vi "test TCX read (installed 71).vi"() -> ()   [LabVIEW 2011] (continued)
ensions></Trackpoint><Trackpoint><Time>2008-03-03T23:23:27Z</Time><Position><LatitudeDegrees>35.882176</LatitudeDegrees><LongitudeDegrees>-78.947276</LongitudeDegrees></Position><AltitudeMeters>80.888</AltitudeMeters><DistanceMeters>20909.645</DistanceMeters><Cadence>83</Cadence><Extensions><TPX xmlns=\"http://www.garmin.com/xmlschemas/ActivityExtension/v2\"><Watts>156</Watts></TPX></Extensions></Trackpoint><Trackpoint><Time>2008-03-03T23:23:28Z</Time><Position><LatitudeDegrees>35.882253</LatitudeDegrees><LongitudeDegrees>-78.947252</LongitudeDegrees></Position><AltitudeMeters>80.888</AltitudeMeters><DistanceMeters>20918.570</DistanceMeters><Cadence>81</Cadence><Extensions><TPX xmlns=\"http://www.garmin.com/xmlschemas/ActivityExtension/v2\"><Watts>129</Watts></TPX></Extensions></Trackpoint><Trackpoint><Time>2008-03-03T23:23:29Z</Time><Position><LatitudeDegrees>35.882330</LatitudeDegrees><LongitudeDegrees>-78.947230</LongitudeDegrees></Position><AltitudeMeters>80.888</AltitudeMeters><DistanceMeters>20927.145</DistanceMeters><Cadence>80</Cadence><Extensions><TPX xmlns=\"http://www.garmin.com/xmlschemas/ActivityExtension/v2\"><Watts>133</Watts></TPX></Extensions></Trackpoint><Trackpoint><Time>2008-03-03T23:23:30Z</Time><Position><LatitudeDegrees>35.882405</LatitudeDegrees><LongitudeDegrees>-78.947209</LongitudeDegrees></Position><AltitudeMeters>81.369</AltitudeMeters><DistanceMeters>20935.766</DistanceMeters><Cadence>79</Cadence><Extensions><TPX xmlns=\"http://www.garmin.com/xmlschemas/ActivityExtension/v2\"><Watts>132</Watts></TPX></Extensions></Trackpoint><Trackpoint><Time>2008-03-03T23:23:31Z</Time><Position><LatitudeDegrees>35.882479</LatitudeDegrees><LongitudeDegrees>-78.947186</LongitudeDegrees></Position><AltitudeMeters>81.369</AltitudeMeters><DistanceMeters>20944.205</DistanceMeters><Cadence>78</Cadence><Extensions><TPX xmlns=\"http://www.garmin.com/xmlschemas/ActivityExtension/v2\"><Watts>147</Watts></TPX></Extensions></Trackpoint><Trackpoint><Time>2008-03-03T23:23:32Z</Time><Position><LatitudeDegrees>35.882553</LatitudeDegrees><LongitudeDegrees>-78.947165</LongitudeDegrees></Position><AltitudeMeters>81.369</AltitudeMeters><DistanceMeters>20952.598</DistanceMeters><Cadence>77</Cadence><Extensions><TPX xmlns=\"http://www.garmin.com/xmlschemas/ActivityExtension/v2\"><Watts>154</Watts></TPX></Extensions></Trackpoint><Trackpoint><Time>2008-03-03T23:23:33Z</Time><Position><LatitudeDegrees>35.882626</LatitudeDegrees><LongitudeDegrees>-78.947144</LongitudeDegrees></Position><AltitudeMeters>81.849</AltitudeMeters><DistanceMeters>20960.939</DistanceMeters><Cadence>77</Cadence><Extensions><TPX xmlns=\"http://www.garmin.com/xmlschemas/ActivityExtension/v2\"><Watts>162</Watts></TPX></Extensions></Trackpoint><Trackpoint><Time>2008-03-03T23:23:34Z</Time><Position><LatitudeDegrees>35.882699</LatitudeDegrees><LongitudeDegrees>-78.947123</LongitudeDegrees></Position><AltitudeMeters>81.849</AltitudeMeters><DistanceMeters>20969.234</DistanceMeters><Cadence>77</Cadence><Extensions><TPX xmlns=\"http://www.garmin.com/xmlschemas/ActivityExtension/v2\"><Watts>162</Watts></TPX></Extensions></Trackpoint><Trackpoint><Time>2008-03-03T23:23:35Z</Time><Position><LatitudeDegrees>35.882771</LatitudeDegrees><LongitudeDegrees>-78.947102</LongitudeDegrees></Position><AltitudeMeters>82.330</AltitudeMeters><DistanceMeters>20977.500</DistanceMeters><Cadence>77</Cadence><Extensions><TPX xmlns=\"http://www.garmin.com/xmlschemas/ActivityExtension/v2\"><Watts>163</Watts></TPX></Extensions></Trackpoint><Trackpoint><Time>2008-03-03T23:23:36Z</Time><Position><LatitudeDegrees>35.882844</LatitudeDegrees><LongitudeDegrees>-78.947082</LongitudeDegrees></Position><AltitudeMeters>82.330</AltitudeMeters><DistanceMeters>20985.758</DistanceMeters><Cadence>77</Cadence><Extensions><TPX xmlns=\"http://www.garmin.com/xmlschemas/ActivityExtension/v2\"><Watts>185</Watts></TPX></Extensions></Trackpoint><Trackpoint><Time>2008-03-03T23:23:37Z</Time><Position><LatitudeDegrees>35.882917</LatitudeDegrees><LongitudeDegrees>-78.947061</LongitudeDegrees></Position><AltitudeMeters>82.330</AltitudeMeters><DistanceMeters>20994.070</DistanceMeters><Cadence>77</Cadence><Extensions><TPX xmlns=\"http://www.garmin.com/xmlschemas/ActivityExtension/v2\"><Watts>195</Watts></TPX></Extensions></Trackpoint><Trackpoint><Time>2008-03-03T23:23:38Z</Time><Position><LatitudeDegrees>35.882990</LatitudeDegrees><LongitudeDegrees>-78.947042</LongitudeDegrees></Position><AltitudeMeters>82.330</AltitudeMeters><DistanceMeters>21002.367</DistanceMeters><Cadence>77</Cadence><Extensions><TPX xmlns=\"http://www.garmin.com/xmlschemas/ActivityExtension/v2\"><Watts>197</Watts></TPX></Extensions></Trackpoint><Trackpoint><Time>2008-03-03T23:23:39Z</Time><Position><LatitudeDegrees>35.883063</LatitudeDegrees><LongitudeDegrees>-78.947023</LongitudeDegrees></Position><AltitudeMeters>82.811</AltitudeMeters><DistanceMeters>21010.590</DistanceMeters><Cadence>77</Cadence><Extensions><TPX xmlns=\"http://www.garmin.com/xmlschemas/ActivityExtension/v2\"><Watts>196</Watts></TPX></Extensions></Trackpoint><Trackpoint><Time>2008-03-03T23:23:40Z</Time><Position><LatitudeDegrees>35.883135</LatitudeDegrees><LongitudeDegrees>-78.947001</LongitudeDegrees></Position><AltitudeMeters>82.811</AltitudeMeters><DistanceMeters>21018.857</DistanceMeters><Cadence>77</Cadence><Extensions><TPX xmlns=\"http://www.garmin.com/xmlschemas/ActivityExtension/v2\"><Watts>185</Watts></TPX></Extensions></Trackpoint><Trackpoint><Time>2008-03-03T23:23:41Z</Time><Position><LatitudeDegrees>35.883208</LatitudeDegrees><LongitudeDegrees>-78.946980</LongitudeDegrees></Position><AltitudeMeters>82.811</AltitudeMeters><DistanceMeters>21027.145</DistanceMeters><Cadence>76</Cadence><Extensions><TPX xmlns=\"http://www.garmin.com/xmlschemas/ActivityExtension/v2\"><Watts>181</Watts></TPX></Extensions></Trackpoint><Trackpoint><Time>2008-03-03T23:23:42Z</Time><Position><LatitudeDegrees>35.883280</LatitudeDegrees><LongitudeDegrees>-78.946958</LongitudeDegrees></Position><AltitudeMeters>82.811</AltitudeMeters><DistanceMeters>21035.389</DistanceMeters><Cadence>76</Cadence><Extensions><TPX xmlns=\"http://www.garmin.com/xmlschemas/ActivityExtension/v2\"><Watts>180</Watts></TPX></Extensions></Trackpoint><Trackpoint><Time>2008-03-03T23:23:43Z</Time><Position><LatitudeDegrees>35.883351</LatitudeDegrees><LongitudeDegrees>-78.946937</LongitudeDegrees></Position><AltitudeMeters>82.811</AltitudeMeters><DistanceMeters>21043.555</DistanceMeters><Cadence>76</Cadence><Extensions><TPX xmlns=\"http://www.garmin.com/xmlschemas/ActivityExtension/v2\"><Watts>159</Watts></TPX></Extensions></Trackpoint><Trackpoint><Time>2008-03-03T23:23:44Z</Time><Position><LatitudeDegrees>35.883423</LatitudeDegrees><LongitudeDegrees>-78.946915</LongitudeDegrees></Position><AltitudeMeters>83.291</AltitudeMeters><DistanceMeters>21051.729</DistanceMeters><Cadence>75</Cadence><Extensions><TPX xmlns=\"http://www.garmin.com/xmlschemas/ActivityExtension/v2\"><Watts>147</Watts></TPX></Extensions></Trackpoint><Trackpoint><Time>2008-03-03T23:23:45Z</Time><Position><LatitudeDegrees>35.883493</LatitudeDegrees><LongitudeDegrees>-78.946891</LongitudeDegrees></Position><AltitudeMeters>83.772</AltitudeMeters><DistanceMeters>21059.771</DistanceMeters><Cadence>74</Cadence><Extensions><TPX xmlns=\"http://www.garmin.com/xmlschemas/ActivityExtension/v2\"><Watts>148</Watts></TPX></Extensions></Trackpoint><Trackpoint><Time>2008-03-03T23:23:46Z</Time><Position><LatitudeDegrees>35.883561</LatitudeDegrees><LongitudeDegrees>-78.946866</LongitudeDegrees></Position><AltitudeMeters>83.291</AltitudeMeters><DistanceMeters>21067.736</DistanceMeters><Cadence>74</Cadence><Extensions><TPX xmlns=\"http://www.garmin.com/xmlschemas/ActivityExtension/v2\"><Watts>158</Watts></TPX></Extensions></Trackpoint><Trackpoint><Time>2008-03-03T23:23:47Z</Time><Position><LatitudeDegrees>35.883629</LatitudeDegrees><LongitudeDegrees>-78.946838</LongitudeDegrees></Position><AltitudeMeters>83.291</AltitudeMeters><DistanceMeters>21075.658</DistanceMeters><Cadence>74</Cadence><Extensions><TPX xmlns=\"http://www.garmin.com/xmlschemas/ActivityExtension/v2\"><Watts>159</Watts></TPX></Extensions></Trackpoint><Trackpoint><Time>2008-03-03T23:23:48Z</Time><Position><LatitudeDegrees>35.883696</LatitudeDegrees><LongitudeDegrees>-78.946808</LongitudeDegrees></Position><AltitudeMeters>83.772</AltitudeMeters><DistanceMeters>21083.572</DistanceMeters><Cadence>73</Cadence><Extensions><TPX xmlns=\"http://www.garmin.com/xmlschemas/ActivityExtension/v2\"><Watts>205</Watts></TPX></Extensions></Trackpoint><Trackpoint><Time>2008-03-03T23:23:49Z</Time><Position><LatitudeDegrees>35.883763</LatitudeDegrees><LongitudeDegrees>-78.946776</LongitudeDegrees></Position><AltitudeMeters>83.291</AltitudeMeters><DistanceMeters>21091.551</DistanceMeters><Cadence>74</Cadence><Extensions><TPX xmlns=\"http://www.garmin.com/xmlschemas/ActivityExtension/v2\"><Watts>230</Watts></TPX></Extensions></Trackpoint><Trackpoint><Time>2008-03-03T23:23:50Z</Time><Position><LatitudeDegrees>35.883829</LatitudeDegrees><LongitudeDegrees>-78.946741</LongitudeDegrees></Position><AltitudeMeters>83.291</AltitudeMeters><DistanceMeters>21099.539</DistanceMeters><Cadence>74</Cadence><Extensions><TPX xmlns=\"http://www.garmin.com/xmlschemas/ActivityExtension/v2\"><Watts>235</Watts></TPX></Extensions></Trackpoint><Trackpoint><Time>2008-03-03T23:23:51Z</Time><Position><LatitudeDegrees>35.883895</LatitudeDegrees><LongitudeDegrees>-78.946704</LongitudeDegrees></Position><AltitudeMeters>83.772</AltitudeMeters><DistanceMeters>21107.541</DistanceMeters><Cadence>74</Cadence><Extensions><TPX xmlns=\"http://www.garmin.com/xmlschemas/ActivityExtension/v2\"><Watts>234</Watts></TPX></Extensions></Trackpoint><Trackpoint><Time>2008-03-03T23:23:52Z</Time><Position><LatitudeDegrees>35.883959</LatitudeDegrees><LongitudeDegrees>-78.946664</LongitudeDegrees></Position><AltitudeMeters>84.253</AltitudeMeters><DistanceMeters>21115.559</DistanceMeters><Cadence>74</Cadence><Extensions><TPX xmlns=\"http://www.garmin.com/xmlschemas/ActivityExtension/v2\"><Watts>217</Watts></TPX></Extensions></Trackpoint><Trackpoint><Time>2008-03-03T23:23:53Z</Time><Position><LatitudeDegrees>35.884022</LatitudeDegrees><LongitudeDegrees>-78.946623</LongitudeDegrees></Position><AltitudeMeters>84.253</AltitudeMeters><DistanceMeters>21123.479</DistanceMeters><Cadence>74</Cadence><Extensions><TPX xmlns=\"http://www.garmin.com/xmlschemas/ActivityExtension/v2\"><Watts>205</Watts></TPX></Extensions></Trackpoint><Trackpoint><Time>2008-03-03T23:23:54Z</Time><Position><LatitudeDegrees>35.884085</LatitudeDegrees><LongitudeDegrees>-78.946579</LongitudeDegrees></Position><AltitudeMeters>84.733</AltitudeMeters><DistanceMeters>21131.467</DistanceMeters><Cadence>74</Cadence><Extensions><TPX xmlns=\"http://www.garmin.com/xmlschemas/ActivityExtension/v2\"><Watts>195</Watts></TPX></Extensions></Trackpoint><Trackpoint><Time>2008-03-03T23:23:55Z</Time><Position><LatitudeDegrees>35.884147</LatitudeDegrees><LongitudeDegrees>-78.946532</LongitudeDegrees></Position><AltitudeMeters>84.733</AltitudeMeters><DistanceMeters>21139.529</DistanceMeters><Cadence>74</Cadence><Extensions><TPX xmlns=\"http://www.garmin.com/xmlschemas/ActivityExtension/v2\"><Watts>184</Watts></TPX></Extensions></Trackpoint><Trackpoint><Time>2008-03-03T23:23:56Z</Time><Position><LatitudeDegrees>35.884208</LatitudeDegrees><LongitudeDegrees>-78.946484</LongitudeDegrees></Position><AltitudeMeters>85.214</AltitudeMeters><DistanceMeters>21147.596</DistanceMeters><Cadence>75</Cadence><Extensions><TPX xmlns=\"http://www.garmin.com/xmlschemas/ActivityExtension/v2\"><Watts>164</Watts></TPX></Extensions></Trackpoint><Trackpoint><Time>2008-03-03T23:23:57Z</Time><Position><LatitudeDegrees>35.884268</LatitudeDegrees><LongitudeDegrees>-78.946432</LongitudeDegrees></Position><AltitudeMeters>85.214</AltitudeMeters><DistanceMeters>21155.812</DistanceMeters><Cadence>76</Cadence><Extensions><TPX xmlns=\"http://www.garmin.com/xmlschemas/ActivityExtension/v2\"><Watts>145</Watts></TPX></Extensions></Trackpoint><Trackpoint><Time>2008-03-03T23:23:58Z</Time><Position><LatitudeDegrees>35.884328</LatitudeDegrees><LongitudeDegrees>-78.946376</LongitudeDegrees></Position><AltitudeMeters>85.214</AltitudeMeters><DistanceMeters>21164.123</DistanceMeters><Cadence>77</Cadence><Extensions><TPX xmlns=\"http://www.garmin.com/xmlschemas/ActivityExtension/v2\"><Watts>110</Watts></TPX></Extensions></Trackpoint><Trackpoint><Time>2008-03-03T23:23:59Z</Time><Position><LatitudeDegrees>35.884389</LatitudeDegrees><LongitudeDegrees>-78.946319</LongitudeDegrees></Position><AltitudeMeters>85.214</AltitudeMeters><DistanceMeters>21172.600</DistanceMeters><Cadence>77</Cadence><Extensions><TPX xmlns=\"http://www.garmin.com/xmlschemas/ActivityExtension/v2\"><Watts>111</Watts></TPX></Extensions></Trackpoint><Trackpoint><Time>2008-03-03T23:24:00Z</Time><Position><LatitudeDegrees>35.884449</LatitudeDegrees><LongitudeDegrees>-78.946261</LongitudeDegrees></Position><AltitudeMeters>85.214</AltitudeMeters><DistanceMeters>21181.143</DistanceMeters><Cadence>78</Cadence><Extensions><TPX xmlns=\"http://www.garmin.com/xmlschemas/ActivityExtension/v2\"><Watts>97</Watts></TPX></Extensions></Trackpoint><Trackpoint><Time>2008-03-03T23:24:01Z</Time><Position><LatitudeDegrees>35.884510</LatitudeDegrees><LongitudeDegrees>-78.946201</LongitudeDegrees></Position><AltitudeMeters>85.214</AltitudeMeters><DistanceMeters>21189.721</DistanceMeters><Cadence>80</Cadence><Extensions><TPX xmlns=\"http://www.garmin.com/xmlschemas/ActivityExtension/v2\"><Watts>98</Watts></TPX></Extensions></Trackpoint><Trackpoint><Time>2008-03-03T23:24:02Z</Time><Position><LatitudeDegrees>35.884571</LatitudeDegrees><LongitudeDegrees>-78.946138</LongitudeDegrees></Position><AltitudeMeters>84.733</AltitudeMeters><DistanceMeters>21198.600</DistanceMeters><Cadence>82</Cadence><Extensions><TPX xmlns=\"http://www.garmin.com/xmlschemas/ActivityExtension/v2\"><Watts>92</Watts></TPX></Extensions></Trackpoint><Trackpoint><Time>2008-03-03T23:24:03Z</Time><Position><LatitudeDegrees>35.884633</LatitudeDegrees><LongitudeDegrees>-78.946075</LongitudeDegrees></Position><AltitudeMeters>84.733</AltitudeMeters><DistanceMeters>21207.596</DistanceMeters><Cadence>85</Cadence><Extensions><TPX xmlns=\"http://www.garmin.com/xmlschemas/ActivityExtension/v2\"><Watts>83</Watts></TPX></Extensions></Trackpoint><Trackpoint><Time>2008-03-03T23:24:04Z</Time><Position><LatitudeDegrees>35.884699</LatitudeDegrees><LongitudeDegrees>-78.946010</LongitudeDegrees></Position><AltitudeMeters>84.253</AltitudeMeters><DistanceMeters>21216.910</DistanceMeters><Cadence>85</Cadence><Extensions><TPX xmlns=\"http://www.garmin.com/xmlschemas/ActivityExtension/v2\"><Watts>82</Watts></TPX></Extensions></Trackpoint><Trackpoint><Time>2008-03-03T23:24:05Z</Time><Position><LatitudeDegrees>35.884764</LatitudeDegrees><LongitudeDegrees>-78.945943</LongitudeDegrees></Position><AltitudeMeters>84.253</AltitudeMeters><DistanceMeters>21226.375</DistanceMeters><Cadence>87</Cadence><Extensions><TPX xmlns=\"http://www.garmin.com/xmlschemas/ActivityExtension/v2\"><Watts>76</Watts></TPX></Extensions></Trackpoint><Trackpoint><Time>2008-03-03T23:24:06Z</Time><Position><LatitudeDegrees>35.884828</LatitudeDegrees><LongitudeDegrees>-78.945874</LongitudeDegrees></Position><AltitudeMeters>84.253</AltitudeMeters><DistanceMeters>21235.848</DistanceMeters><Cadence>87</Cadence><Extensions><TPX xmlns=\"http://www.garmin.com/xmlschemas/ActivityExtension/v2\"><Watts>83</Watts></TPX></Extensions></Trackpoint><Trackpoint><Time>2008-03-03T23:24:07Z</Time><Position><LatitudeDegrees>35.884893</LatitudeDegrees><LongitudeDegrees>-78.945806</LongitudeDegrees></Position><AltitudeMeters>83.772</AltitudeMeters><DistanceMeters>21245.301</DistanceMeters><Cadence>87</Cadence><Extensions><TPX xmlns=\"http://www.garmin.com/xmlschemas/ActivityExtension/v2\"><Watts>95</Watts></TPX></Extensions></Trackpoint><Trackpoint><Time>2008-03-03T23:24:08Z</Time><Position><LatitudeDegrees>35.884958</LatitudeDegrees><LongitudeDegrees>-78.945738</LongitudeDegrees></Position><AltitudeMeters>83.291</AltitudeMeters><DistanceMeters>21254.760</DistanceMeters><Cadence>88</Cadence><Extensions><TPX xmlns=\"http://www.garmin.com/xmlschemas/ActivityExtension/v2\"><Watts>133</Watts></TPX></Extensions></Trackpoint><Trackpoint><Time>2008-03-03T23:24:09Z</Time><Position><LatitudeDegrees>35.885023</LatitudeDegrees><LongitudeDegrees>-78.945671</LongitudeDegrees></Position><AltitudeMeters>83.291</AltitudeMeters><DistanceMeters>21264.236</DistanceMeters><Cadence>88</Cadence><Extensions><TPX xmlns=\"http://www.garmin.com/xmlschemas/ActivityExtension/v2\"><Watts>134</Watts></TPX></Extensions></Trackpoint><Trackpoint><Time>2008-03-03T23:24:10Z</Time><Position><LatitudeDegrees>35.885089</LatitudeDegrees><LongitudeDegrees>-78.945603</LongitudeDegrees></Position><AltitudeMeters>83.772</AltitudeMeters><DistanceMeters>21273.727</DistanceMeters><Cadence>87</Cadence><Extensions><TPX xmlns=\"http://www.garmin.com/xmlschemas/ActivityExtension/v2\"><Watts>139</Watts></TPX></Extensions></Trackpoint><Trackpoint><Time>2008-03-03T23:24:11Z</Time><Position><LatitudeDegrees>35.885154</LatitudeDegrees><LongitudeDegrees>-78.945536</LongitudeDegrees></Position><AltitudeMeters>83.772</AltitudeMeters><DistanceMeters>21283.127</DistanceMeters><Cadence>86</Cadence><Extensions><TPX xmlns=\"http://www.garmin.com/xmlschemas/ActivityExtension/v2\"><Watts>133</Watts></TPX></Extensions></Trackpoint><Trackpoint><Time>2008-03-03T23:24:12Z</Time><Position><LatitudeDegrees>35.885218</LatitudeDegrees><LongitudeDegrees>-78.945470</LongitudeDegrees></Position><AltitudeMeters>83.772</AltitudeMeters><DistanceMeters>21292.441</DistanceMeters><Cadence>86</Cadence><Extensions><TPX xmlns=\"http://www.garmin.com/xmlschemas/ActivityExtension/v2\"><Watts>132</Watts></TPX></Extensions></Trackpoint><Trackpoint><Time>2008-03-03T23:24:13Z</Time><Position><LatitudeDegrees>35.885284</LatitudeDegrees><LongitudeDegrees>-78.945405</LongitudeDegrees></Position><AltitudeMeters>83.772</AltitudeMeters><DistanceMeters>21301.773</DistanceMeters><Cadence>87</Cadence><Extensions><TPX xmlns=\"http://www.garmin.com/xmlschemas/ActivityExtension/v2\"><Watts>184</Watts></TPX></Extensions></Trackpoint><Trackpoint><Time>2008-03-03T23:24:14Z</Time><Position><LatitudeDegrees>35.885350</LatitudeDegrees><LongitudeDegrees>-78.945340</LongitudeDegrees></Position><AltitudeMeters>83.772</AltitudeMeters><DistanceMeters>21311.172</DistanceMeters><Cadence>87</Cadence><Extensions><TPX xmlns=\"http://www.garmin.com/xmlschemas/ActivityExtension/v2\"><Watts>263</Watts></TPX></Extensions></Trackpoint><Trackpoint><Time>2008-03-03T23:24:15Z</Time><Position><LatitudeDegrees>35.885415</LatitudeDegrees><LongitudeDegrees>-78.945274</LongitudeDegrees></Position><AltitudeMeters>83.772</AltitudeMeters><DistanceMeters>21320.535</DistanceMeters><Cadence>86</Cadence><Extensions><TPX xmlns=\"http://www.garmin.com/xmlschemas/ActivityExtension/v2\"><Watts>270</Watts></TPX></Extensions></Trackpoint><Trackpoint><Time>2008-03-03T23:24:16Z</Time><Position><LatitudeDegrees>35.885479</LatitudeDegrees><LongitudeDegrees>-78.945208</LongitudeDegrees></Position><AltitudeMeters>84.253</AltitudeMeters><DistanceMeters>21329.799</DistanceMeters><Cadence>86</Cadence><Extensions><TPX xmlns=\"http://www.garmin.com/xmlschemas/ActivityExtension/v2\"><Watts>268</Watts></TPX></Extensions></Trackpoint><Trackpoint><Time>2008-03-03T23:24:17Z</Time><Position><LatitudeDegrees>35.885542</LatitudeDegrees><LongitudeDegrees>-78.945140</LongitudeDegrees></Position><AltitudeMeters>84.733</AltitudeMeters><DistanceMeters>21339.119</DistanceMeters><Cadence>86</Cadence><Extensions><TPX xmlns=\"http://www.garmin.com/xmlschemas/ActivityExtension/v2\"><Watts>258</Watts></TPX></Extensions></Trackpoint><Trackpoint><Time>2008-03-03T23:24:18Z</Time><Position><LatitudeDegrees>35.885605</LatitudeDegrees><LongitudeDegrees>-78.945072</LongitudeDegrees></Position><AltitudeMeters>84.733</AltitudeMeters><DistanceMeters>21348.438</DistanceMeters><Cadence>86</Cadence><Extensions><TPX xmlns=\"http://www.garmin.com/xmlschemas/ActivityExtension/v2\"><Watts>263</Watts></TPX></Extensions></Trackpoint><Trackpoint><Time>2008-03-03T23:24:19Z</Time><Position><LatitudeDegrees>35.885670</LatitudeDegrees><LongitudeDegrees>-78.945004</LongitudeDegrees></Position><AltitudeMeters>85.214</AltitudeMeters><DistanceMeters>21357.840</DistanceMeters><Cadence>86</Cadence><Extensions><TPX xmlns=\"http://www.garmin.com/xmlschemas/ActivityExtension/v2\"><Watts>263</Watts></TPX></Extensions></Trackpoint><Trackpoint><Time>2008-03-03T23:24:20Z</Time><Position><LatitudeDegrees>35.885735</LatitudeDegrees><LongitudeDegrees>-78.944938</LongitudeDegrees></Position><AltitudeMeters>85.695</AltitudeMeters><DistanceMeters>21367.240</DistanceMeters><Cadence>87</Cadence><Extensions><TPX xmlns=\"http://www.garmin.com/xmlschemas/ActivityExtension/v2\"><Watts>283</Watts></TPX></Extensions></Trackpoint><Trackpoint><Time>2008-03-03T23:24:21Z</Time><Position><LatitudeDegrees>35.885800</LatitudeDegrees><LongitudeDegrees>-78.944872</LongitudeDegrees></Position><AltitudeMeters>86.175</AltitudeMeters><DistanceMeters>21376.639</DistanceMeters><Cadence>86</Cadence><Extensions><TPX xmlns=\"http://www.garmin.com/xmlschemas/ActivityExtension/v2\"><Watts>281</Watts></TPX></Extensions></Trackpoint><Trackpoint><Time>2008-03-03T23:24:22Z</Time><Position><LatitudeDegrees>35.885866</LatitudeDegrees><LongitudeDegrees>-78.944809</LongitudeDegrees></Position><AltitudeMeters>86.175</AltitudeMeters><DistanceMeters>21385.852</DistanceMeters><Cadence>85</Cadence><Extensions><TPX xmlns=\"http://www.garmin.com/xmlschemas/ActivityExtension/v2\"><Watts>265</Watts></TPX></Extensions></Trackpoint><Trackpoint><Time>2008-03-03T23:24:23Z</Time><Position><LatitudeDegrees>35.885930</LatitudeDegrees><LongitudeDegrees>-78.944748</LongitudeDegrees></Position><AltitudeMeters>85.695</AltitudeMeters><DistanceMeters>21394.875</DistanceMeters><Cadence>83</Cadence><Extensions><TPX xmlns=\"http://www.garmin.com/xmlschemas/ActivityExtension/v2\"><Watts>180</Watts></TPX></Extensions></Trackpoint><Trackpoint><Time>2008-03-03T23:24:24Z</Time><Position><LatitudeDegrees>35.885996</LatitudeDegrees><LongitudeDegrees>-78.944689</LongitudeDegrees></Position><AltitudeMeters>85.695</AltitudeMeters><DistanceMeters>21403.871</DistanceMeters><Cadence>83</Cadence><Extensions><TPX xmlns=\"http://www.garmin.com/xmlschemas/ActivityExtension/v2\"><Watts>179</Watts></TPX></Extensions></Trackpoint><Trackpoint><Time>2008-03-03T23:24:25Z</Time><Position><LatitudeDegrees>35.886062</LatitudeDegrees><LongitudeDegrees>-78.944634</LongitudeDegrees></Position><AltitudeMeters>85.695</AltitudeMeters><DistanceMeters>21412.711</DistanceMeters><Cadence>81</Cadence><Extensions><TPX xmlns=\"http://www.garmin.com/xmlschemas/ActivityExtension/v2\"><Watts>164</Watts></TPX></Extensions></Trackpoint><Trackpoint><Time>2008-03-03T23:24:26Z</Time><Position><LatitudeDegrees>35.886128</LatitudeDegrees><LongitudeDegrees>-78.944583</LongitudeDegrees></Position><AltitudeMeters>85.695</AltitudeMeters><DistanceMeters>21421.385</DistanceMeters><Cadence>80</Cadence><Extensions><TPX xmlns=\"http://www.garmin.com/xmlschemas/ActivityExtension/v2\"><Watts>154</Watts></TPX></Extensions></Trackpoint><Trackpoint><Time>2008-03-03T23:24:27Z</Time><Position><LatitudeDegrees>35.886195</LatitudeDegrees><LongitudeDegrees>-78.944536</LongitudeDegrees></Position><AltitudeMeters>85.695</AltitudeMeters><DistanceMeters>21429.920</DistanceMeters><Cadence>78</Cadence><Extensions><TPX xmlns=\"http://www.garmin.com/xmlschemas/ActivityExtension/v2\"><Watts>153</Watts></TPX></Extensions></Trackpoint><Trackpoint><Time>2008-03-03T23:24:28Z</Time><Position><LatitudeDegrees>35.886263</LatitudeDegrees><LongitudeDegrees>-78.944493</LongitudeDegrees></Position><AltitudeMeters>85.695</AltitudeMeters><DistanceMeters>21438.398</DistanceMeters><Cadence>78</Cadence><Extensions><TPX xmlns=\"http://www.garmin.com/xmlschemas/ActivityExtension/v2\"><Watts>150</Watts></TPX></Extensions></Trackpoint><Trackpoint><Time>2008-03-03T23:24:29Z</Time><Position><LatitudeDegrees>35.886333</LatitudeDegrees><LongitudeDegrees>-78.944455</LongitudeDegrees></Position><AltitudeMeters>85.695</AltitudeMeters><DistanceMeters>21446.896</DistanceMeters><Cadence>79</Cadence><Extensions><TPX xmlns=\"http://www.garmin.com/xmlschemas/ActivityExtension/v2\"><Watts>130</Watts></TPX></Extensions></Trackpoint><Trackpoint><Time>2008-03-03T23:24:30Z</Time><Position><LatitudeDegrees>35.886404</LatitudeDegrees><LongitudeDegrees>-78.944421</LongitudeDegrees></Position><AltitudeMeters>86.175</AltitudeMeters><DistanceMeters>21455.379</DistanceMeters><Cadence>78</Cadence><Extensions><TPX xmlns=\"http://www.garmin.com/xmlschemas/ActivityExtension/v2\"><Watts>114</Watts></TPX></Extensions></Trackpoint><Trackpoint><Time>2008-03-03T23:24:31Z</Time><Position><LatitudeDegrees>35.886477</LatitudeDegrees><LongitudeDegrees>-78.944391</LongitudeDegrees></Position><AltitudeMeters>85.695</AltitudeMeters><DistanceMeters>21463.840</DistanceMeters><Cadence>78</Cadence><Extensions><TPX xmlns=\"http://www.garmin.com/xmlschemas/ActivityExtension/v2\"><Watts>103</Watts></TPX></Extensions></Trackpoint><Trackpoint><Time>2008-03-03T23:24:32Z</Time><Position><LatitudeDegrees>35.886551</LatitudeDegrees><LongitudeDegrees>-78.944364</LongitudeDegrees></Position><AltitudeMeters>85.695</AltitudeMeters><DistanceMeters>21472.439</DistanceMeters><Cadence>79</Cadence><Extensions><TPX xmlns=\"http://www.garmin.com/xmlschemas/ActivityExtension/v2\"><Watts>103</Watts></TPX></Extensions></Trackpoint><Trackpoint><Time>2008-03-03T23:24:33Z</Time><Position><LatitudeDegrees>35.886626</LatitudeDegrees><LongitudeDegrees>-78.944337</LongitudeDegrees></Position><AltitudeMeters>85.214</AltitudeMeters><DistanceMeters>21481.201</DistanceMeters><Cadence>72</Cadence><Extensions><TPX xmlns=\"http://www.garmin.com/xmlschemas/ActivityExtension/v2\"><Watts>97</Watts></TPX></Extensions></Trackpoint><Trackpoint><Time>2008-03-03T23:24:34Z</Time><Position><LatitudeDegrees>35.886704</LatitudeDegrees><LongitudeDegrees>-78.944310</LongitudeDegrees></Position><AltitudeMeters>85.214</AltitudeMeters><DistanceMeters>21490.156</DistanceMeters><Cadence>74</Cadence><Extensions><TPX xmlns=\"http://www.garmin.com/xmlschemas/ActivityExtension/v2\"><Watts>113</Watts></TPX></Extensions></Trackpoint><Trackpoint><Time>2008-03-03T23:24:35Z</Time><Position><LatitudeDegrees>35.886784</LatitudeDegrees><LongitudeDegrees>-78.944284</LongitudeDegrees></Position><AltitudeMeters>85.214</AltitudeMeters><DistanceMeters>21499.391</DistanceMeters><Cadence>76</Cadence><Extensions><TPX xmlns=\"http://www.garmin.com/xmlschemas/ActivityExtension/v2\"><Watts>114</Watts></TPX></Extensions></Trackpoint><Trackpoint><Time>2008-03-03T23:24:36Z</Time><Position><LatitudeDegrees>35.886867</LatitudeDegrees><LongitudeDegrees>-78.944256</LongitudeDegrees></Position><AltitudeMeters>84.733</AltitudeMeters><DistanceMeters>21508.889</DistanceMeters><Cadence>78</Cadence><Extensions><TPX xmlns=\"http://www.garmin.com/xmlschemas/ActivityExtension/v2\"><Watts>115</Watts></TPX></Extensions></Trackpoint><Trackpoint><Time>2008-03-03T23:24:37Z</Time><Position><LatitudeDegrees>35.886951</LatitudeDegrees><LongitudeDegrees>-78.944226</LongitudeDegrees></Position><AltitudeMeters>84.733</AltitudeMeters><DistanceMeters>21518.637</DistanceMeters><Cadence>67</Cadence><Extensions><TPX xmlns=\"http://www.garmin.com/xmlschemas/ActivityExtension/v2\"><Watts>77</Watts></TPX></Extensions></Trackpoint><Trackpoint><Time>2008-03-03T23:24:38Z</Time><Position><LatitudeDegrees>35.887037</LatitudeDegrees><LongitudeDegrees>-78.944197</LongitudeDegrees></Position><AltitudeMeters>84.733</AltitudeMeters><DistanceMeters>21528.494</DistanceMeters><Cadence>67</Cadence><Extensions><TPX xmlns=\"http://www.garmin.com/xmlschemas/ActivityExtension/v2\"><Watts>78</Watts></TPX></Extensions></Trackpoint><Trackpoint><Time>2008-03-03T23:24:39Z</Time><Position><LatitudeDegrees>35.887126</LatitudeDegrees><LongitudeDegrees>-78.944186</LongitudeDegrees></Position><AltitudeMeters>84.733</AltitudeMeters><DistanceMeters>21538.449</DistanceMeters><Cadence>61</Cadence><Extensions><TPX xmlns=\"http://www.garmin.com/xmlschemas/ActivityExtension/v2\"><Watts>69</Watts></TPX></Extensions></Trackpoint><Trackpoint><Time>2008-03-03T23:24:40Z</Time><Position><LatitudeDegrees>35.887223</LatitudeDegrees><LongitudeDegrees>-78.944237</LongitudeDegrees></Position><AltitudeMeters>84.733</AltitudeMeters><DistanceMeters>21550.215</DistanceMeters><Cadence>61</Cadence><Extensions><TPX xmlns=\"http://www.garmin.com/xmlschemas/ActivityExtension/v2\"><Watts>69</Watts></TPX></Extensions></Trackpoint><Trackpoint><Time>2008-03-03T23:24:41Z</Time><Position><LatitudeDegrees>35.887305</LatitudeDegrees><LongitudeDegrees>-78.944319</LongitudeDegrees></Position><AltitudeMeters>84.253</AltitudeMeters><DistanceMeters>21561.879</DistanceMeters><Cadence>65</Cadence><Extensions><TPX xmlns=\"http://www.garmin.com/xmlschemas/ActivityExtension/v2\"><Watts>92</Watts></TPX></Extensions></Trackpoint><Trackpoint><Time>2008-03-03T23:24:42Z</Time><Position><LatitudeDegrees>35.887353</LatitudeDegrees><LongitudeDegrees>-78.944435</LongitudeDegrees></Position><AltitudeMeters>84.253</AltitudeMeters><DistanceMeters>21573.764</DistanceMeters><Cadence>66</Cadence><Extensions><TPX xmlns=\"http://www.garmin.com/xmlschemas/ActivityExtension/v2\"><Watts>111</Watts></TPX></Extensions></Trackpoint><Trackpoint><Time>2008-03-03T23:24:43Z</Time><Position><LatitudeDegrees>35.887385</LatitudeDegrees><LongitudeDegrees>-78.944552</LongitudeDegrees></Position><AltitudeMeters>82.811</AltitudeMeters><DistanceMeters>21584.902</DistanceMeters><Cadence>66</Cadence><Extensions><TPX xmlns=\"http://www.garmin.com/xmlschemas/ActivityExtension/v2\"><Watts>154</Watts></TPX></Extensions></Trackpoint><Trackpoint><Time>2008-03-03T23:24:44Z</Time><Position><LatitudeDegrees>35.887402</LatitudeDegrees><LongitudeDegrees>-78.944677</LongitudeDegrees></Position><AltitudeMeters>82.811</AltitudeMeters><DistanceMeters>21596.406</DistanceMeters><Cadence>69</Cadence><Extensions><TPX xmlns=\"http://www.garmin.com/xmlschemas/ActivityExtension/v2\"><Watts>230</Watts></TPX></Extensions></Trackpoint><Trackpoint><Time>2008-03-03T23:24:45Z</Time><Position><LatitudeDegrees>35.887414</LatitudeDegrees><LongitudeDegrees>-78.944808</LongitudeDegrees></Position><AltitudeMeters>83.291</AltitudeMeters><DistanceMeters>21608.266</DistanceMeters><Cadence>71</Cadence><Extensions><TPX xmlns=\"http://www.garmin.com/xmlschemas/ActivityExtension/v2\"><Watts>300</Watts></TPX></Extensions></Trackpoint><Trackpoint><Time>2008-03-03T23:24:46Z</Time><Position><LatitudeDegrees>35.887423</LatitudeDegrees><LongitudeDegrees>-78.944941</LongitudeDegrees></Position><AltitudeMeters>82.330</AltitudeMeters><DistanceMeters>21620.381</DistanceMeters><Cadence>72</Cadence><Extensions><TPX xmlns=\"http://www.garmin.com/xmlschemas/ActivityExtension/v2\"><Watts>336</Watts></TPX></Extensions></Trackpoint><Trackpoint><Time>2008-03-03T23:24:47Z</Time><Position><LatitudeDegrees>35.887426</LatitudeDegrees><LongitudeDegrees>-78.945076</LongitudeDegrees></Position><AltitudeMeters>81.849</AltitudeMeters><DistanceMeters>21632.525</DistanceMeters><Cadence>72</Cadence><Extensions><TPX xmlns=\"http://www.garmin.com/xmlschemas/ActivityExtension/v2\"><Watts>423</Watts></TPX></Extensions></Trackpoint><Trackpoint><Time>2008-03-03T23:24:48Z</Time><Position><LatitudeDegrees>35.887433</LatitudeDegrees><LongitudeDegrees>-78.945212</LongitudeDegrees></Position><AltitudeMeters>82.330</AltitudeMeters><DistanceMeters>21644.840</DistanceMeters><Cadence>72</Cadence><Extensions><TPX xmlns=\"http://www.garmin.com/xmlschemas/ActivityExtension/v2\"><Watts>418</Watts></TPX></Extensions></Trackpoint><Trackpoint><Time>2008-03-03T23:24:49Z</Time><Position><LatitudeDegrees>35.887438</LatitudeDegrees><LongitudeDegrees>-78.945343</LongitudeDegrees></Position><AltitudeMeters>82.330</AltitudeMeters><DistanceMeters>21656.609</DistanceMeters><Cadence>71</Cadence><Extensions><TPX xmlns=\"http://www.garmin.com/xmlschemas/ActivityExtension/v2\"><Watts>427</Watts></TPX></Extensions></Trackpoint><Trackpoint><Time>2008-03-03T23:24:50Z</Time><Position><LatitudeDegrees>35.887445</LatitudeDegrees><LongitudeDegrees>-78.945471</LongitudeDegrees></Position><AltitudeMeters>82.330</AltitudeMeters><DistanceMeters>21668.293</DistanceMeters><Cadence>70</Cadence><Extensions><TPX xmlns=\"http://www.garmin.com/xmlschemas/ActivityExtension/v2\"><Watts>441</Watts></TPX></Extensions></Trackpoint><Trackpoint><Time>2008-03-03T23:24:51Z</Time><Position><LatitudeDegrees>35.887447</LatitudeDegrees><LongitudeDegrees>-78.945599</LongitudeDegrees></Position><AltitudeMeters>82.330</AltitudeMeters><DistanceMeters>21679.818</DistanceMeters><Cadence>70</Cadence><Extensions><TPX xmlns=\"http://www.garmin.com/xmlschemas/ActivityExtension/v2\"><Watts>468</Watts></TPX></Extensions></Trackpoint><Trackpoint><Time>2008-03-03T23:24:52Z</Time><Position><LatitudeDegrees>35.887441</LatitudeDegrees><LongitudeDegrees>-78.945726</LongitudeDegrees></Position><AltitudeMeters>82.811</AltitudeMeters><DistanceMeters>21691.289</DistanceMeters><Cadence>68</Cadence><Extensions><TPX xmlns=\"http://www.garmin.com/xmlschemas/ActivityExtension/v2\"><Watts>462</Watts></TPX></Extensions></Trackpoint><Trackpoint><Time>2008-03-03T23:24:53Z</Time><Position><LatitudeDegrees>35.887430</LatitudeDegrees><LongitudeDegrees>-78.945851</LongitudeDegrees></Position><AltitudeMeters>83.291</AltitudeMeters><DistanceMeters>21702.605</DistanceMeters><Cadence>68</Cadence><Extensions><TPX xmlns=\"http://www.garmin.com/xmlschemas/ActivityExtension/v2\"><Watts>464</Watts></TPX></Extensions></Trackpoint><Trackpoint><Time>2008-03-03T23:24:54Z</Time><Position><LatitudeDegrees>35.887416</LatitudeDegrees><LongitudeDegrees>-78.945975</LongitudeDegrees></Position><AltitudeMeters>82.811</AltitudeMeters><DistanceMeters>21713.875</DistanceMeters><Cadence>68</Cadence><Extensions><TPX xmlns=\"http://www.garmin.com/xmlschemas/ActivityExtension/v2\"><Watts>410</Watts></TPX></Extensions></Trackpoint><Trackpoint><Time>2008-03-03T23:24:55Z</Time><Position><LatitudeDegrees>35.887405</LatitudeDegrees><LongitudeDegrees>-78.946099</LongitudeDegrees></Position><AltitudeMeters>82.811</AltitudeMeters><DistanceMeters>21725.260</DistanceMeters><Cadence>68</Cadence><Extensions><TPX xmlns=\"http://www.garmin.com/xmlschemas/ActivityExtension/v2\"><Watts>397</Watts></TPX></Extensions></Trackpoint><Trackpoint><Time>2008-03-03T23:24:56Z</Time><Position><LatitudeDegrees>35.887405</LatitudeDegrees><LongitudeDegrees>-78.946226</LongitudeDegrees></Position><AltitudeMeters>82.330</AltitudeMeters><DistanceMeters>21736.656</DistanceMeters><Cadence>69</Cadence><Extensions><TPX xmlns=\"http://www.garmin.com/xmlschemas/ActivityExtension/v2\"><Watts>394</Watts></TPX></Extensions></Trackpoint><Trackpoint><Time>2008-03-03T23:24:57Z</Time><Position><LatitudeDegrees>35.887419</LatitudeDegrees><LongitudeDegrees>-78.946355</LongitudeDegrees></Position><AltitudeMeters>82.330</AltitudeMeters><DistanceMeters>21748.424</DistanceMeters><Cadence>71</Cadence><Extensions><TPX xmlns=\"http://www.garmin.com/xmlschemas/ActivityExtension/v2\"><Watts>391</Watts></TPX></Extensions></Trackpoint><Trackpoint><Time>2008-03-03T23:24:58Z</Time><Position><LatitudeDegrees>35.887433</LatitudeDegrees><LongitudeDegrees>-78.946485</LongitudeDegrees></Position><AltitudeMeters>81.849</AltitudeMeters><DistanceMeters>21760.285</DistanceMeters><Cadence>72</Cadence><Extensions><TPX xmlns=\"http://www.garmin.com/xmlschemas/ActivityExtension/v2\"><Watts>391</Watts></TPX></Extensions></Trackpoint><Trackpoint><Time>2008-03-03T23:24:59Z</Time><Position><LatitudeDegrees>35.887440</LatitudeDegrees><LongitudeDegrees>-78.946617</LongitudeDegrees></Position><AltitudeMeters>81.849</AltitudeMeters><DistanceMeters>21772.211</DistanceMeters><Cadence>72</Cadence><Extensions><TPX xmlns=\"http://www.garmin.com/xmlschemas/ActivityExtension/v2\"><Watts>360</Watts></TPX></Extensions></Trackpoint><Trackpoint><Time>2008-03-03T23:25:00Z</Time><Position><LatitudeDegrees>35.887459</LatitudeDegrees><LongitudeDegrees>-78.946747</LongitudeDegrees></Position><AltitudeMeters>81.369</AltitudeMeters><DistanceMeters>21784.115</DistanceMeters><Cadence>72</Cadence><Extensions><TPX xmlns=\"http://www.garmin.com/xmlschemas/ActivityExtension/v2\"><Watts>355</Watts></TPX></Extensions></Trackpoint><Trackpoint><Time>2008-03-03T23:25:01Z</Time><Position><LatitudeDegrees>35.887494</LatitudeDegrees><LongitudeDegrees>-78.946873</LongitudeDegrees></Position><AltitudeMeters>81.849</AltitudeMeters><DistanceMeters>21796.094</DistanceMeters><Cadence>73</Cadence><Extensions><TPX xmlns=\"http://www.garmin.com/xmlschemas/ActivityExtension/v2\"><Watts>359</Watts></TPX></Extensions></Trackpoint><Trackpoint><Time>2008-03-03T23:25:02Z</Time><Position><LatitudeDegrees>35.887539</LatitudeDegrees><LongitudeDegrees>-78.947000</LongitudeDegrees></Position><AltitudeMeters>81.849</AltitudeMeters><DistanceMeters>21808.664</DistanceMeters><Cadence>75</Cadence><Extensions><TPX xmlns=\"http://www.garmin.com/xmlschemas/ActivityExtension/v2\"><Watts>355</Watts></TPX></Extensions></Trackpoint><Trackpoint><Time>2008-03-03T23:25:03Z</Time><Position><LatitudeDegrees>35.887590</LatitudeDegrees><LongitudeDegrees>-78.947128</LongitudeDegrees></Position><AltitudeMeters>80.888</AltitudeMeters><DistanceMeters>21821.500</DistanceMeters><Cadence>75</Cadence><Extensions><TPX xmlns=\"http://www.garmin.com/xmlschemas/ActivityExtension/v2\"><Watts>322</Watts></TPX></Extensions></Trackpoint><Trackpoint><Time>2008-03-03T23:25:04Z</Time><Position><LatitudeDegrees>35.887641</LatitudeDegrees><LongitudeDegrees>-78.947258</LongitudeDegrees></Position><AltitudeMeters>80.407</AltitudeMeters><DistanceMeters>21834.566</DistanceMeters><Cadence>78</Cadence><Extensions><TPX xmlns=\"http://www.garmin.com/xmlschemas/ActivityExtension/v2\"><Watts>118</Watts></TPX></Extensions></Trackpoint><Trackpoint><Time>2008-03-03T23:25:05Z</Time><Position><LatitudeDegrees>35.887687</LatitudeDegrees><LongitudeDegrees>-78.947394</LongitudeDegrees></Position><AltitudeMeters>79.927</AltitudeMeters><DistanceMeters>21847.883</DistanceMeters><Cadence>80</Cadence><Extensions><TPX xmlns=\"http://www.garmin.com/xmlschemas/ActivityExtension/v2\"><Watts>80</Watts></TPX></Extensions></Trackpoint><Trackpoint><Time>2008-03-03T23:25:06Z</Time><Position><LatitudeDegrees>35.887732</LatitudeDegrees><LongitudeDegrees>-78.947534</LongitudeDegrees></Position><AltitudeMeters>78.965</AltitudeMeters><DistanceMeters>21861.508</DistanceMeters><Cadence>82</Cadence><Extensions><TPX xmlns=\"http://www.garmin.com/xmlschemas/ActivityExtension/v2\"><Watts>54</Watts></TPX></Extensions></Trackpoint><Trackpoint><Time>2008-03-03T23:25:07Z</Time><Position><LatitudeDegrees>35.887781</LatitudeDegrees><LongitudeDegrees>-78.947676</LongitudeDegrees></Position><AltitudeMeters>78.004</AltitudeMeters><DistanceMeters>21875.385</DistanceMeters><Cadence>84</Cadence><Extensions><TPX xmlns=\"http://www.garmin.com/xmlschemas/ActivityExtension/v2\"><Watts>54</Watts></TPX></Extensions></Trackpoint><Trackpoint><Time>2008-03-03T23:25:08Z</Time><Position><LatitudeDegrees>35.887838</LatitudeDegrees><LongitudeDegrees>-78.947817</LongitudeDegrees></Position><AltitudeMeters>77.043</AltitudeMeters><DistanceMeters>21889.635</DistanceMeters><Cadence>85</Cadence><Extensions><TPX xmlns=\"http://www.garmin.com/xmlschemas/ActivityExtension/v2\"><Watts>63</Watts></TPX></Extensions></Trackpoint><Trackpoint><Time>2008-03-03T23:25:09Z</Time><Position><LatitudeDegrees>35.887898</LatitudeDegrees><LongitudeDegrees>-78.947960</LongitudeDegrees></Position><AltitudeMeters>75.601</AltitudeMeters><DistanceMeters>21904.141</DistanceMeters><Cadence>87</Cadence><Extensions><TPX 
